vi "Read Port1.vi"(8 "error in (no error)":errorcluster, 11 "MPU in":refnum<class "MPU.lvclass">) -> (0 "error out":errorcluster, 3 "MPU out":refnum<class "MPU.lvclass">)   [LabVIEW 2018]
uses:
  <vilib>/eio/EIOMethodNode/EIOMethodNode.xnode
  <vilib>/rvi/eio/common/nirviEmuTemplateMethod_errors.vi
  MPU.lvclass
panel:
  out "Timeouted":bool
  in  "Timeout":i16
  out "Data":u8
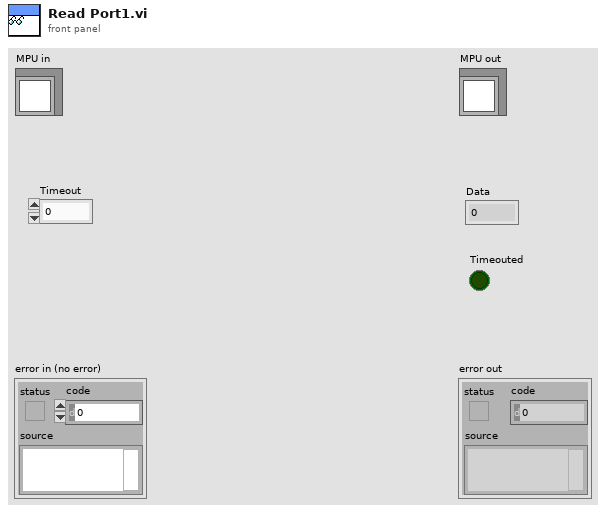
[diagram p1: front panel]
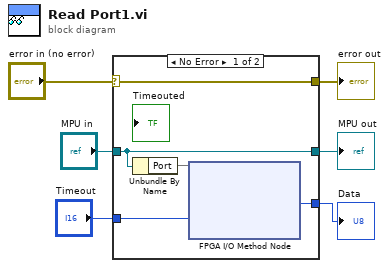
[diagram p0: block diagram]
diagram:
  n1 = case shown="No Error" "error in (no error)" {
    selector: "error in (no error)" -> [w11 w12]
    tunnel: [w11 w12] -> w5
    tunnel: [w10 w13] -> w3
    tunnel: "MPU in" -> [w10 w13]
    tunnel: "Timeout" -> [w8 _]
    tunnel: [w7 _] -> w1
    frame No Error {
      n2 = Unbundle By Name(w10) -> ("Port"=w9)
      n3 = xnode "FPGA I/O Method Node"("FPGA I/O In"=w9, "Timeout (ms)"=w8) -> ("Data"=w7:u8)  [unwired: 2 out]
    }
    frame Error {
    }
  }
  "error out" <- w5
  "MPU out" <- w3
  "Data" <- w1
